vi "SiPM_IV_Tests.vi"(0 "Nb of Pixels":u16, 2 "SiPM Model":string="Hamamatsu_", 3 "SiPM Supplier":string="Hamamatsu_", 4 "Save Reults to file":bool, 5 "Specify folder to save results":path=path "C:/Users/John/Desktop/RESULTS") -> ()   [LabVIEW 2015]
uses:
  <vilib>/Utility/file.llb/Write Delimited Spreadsheet (string).vi
  <vilib>/Utility/file.llb/Write Delimited Spreadsheet (DBL).vi
  <vilib>/Analysis/NI_AALPro.lvlib
panel:
  out "Quenching Resistance":dbl format="%#.3p"
  in  "Process Stop Button":bool
  in  "Read\nTemperature":bool
  in  "Load file":bool
  out "Meassurement \n   In Progress":bool
  out "BIAS Voltage":dbl
  out "Resistance (Overall)":dbl format="%#.3p"
  in  "Start IV":bool
  in  "Current Limit (A)":dbl=0.5
  in  "Enable Time Delay":bool=TRUE
  in  "Time Delay (s)":dbl=1.0
  in  "Nb of Steps":dbl
  in  "Step size (V)":dbl
  in  "Starting Voltage (V)":dbl
  out "I-V graph":cluster{dbl[], "Best Linear Fit":dbl[]}[](graph)
  out "Current Chart":dbl(graph)
  out "Temperature":dbl(slide) scale=0.0..30.0
  in  "Initial Range":dbl=2e-06 min=2e-11 max=0.02 format="%.2e"
  in  "V-Source Range (100:0)":u16(ring)=1 items=["+/- 100 Volts", "+/- 1000 Volts"]
  # "NCSR  DEMOKRITOS\nInstitute of Nuclear and Particle Physics\nDetectors Instrumentation Laboratory"
  # "Si PhotoMultiplier  I-V Measurements"
  # "Device Under Test Type"
  # "Measurement Parameters"
  # "Keithley 6517A"
  # "Additional Parameters"
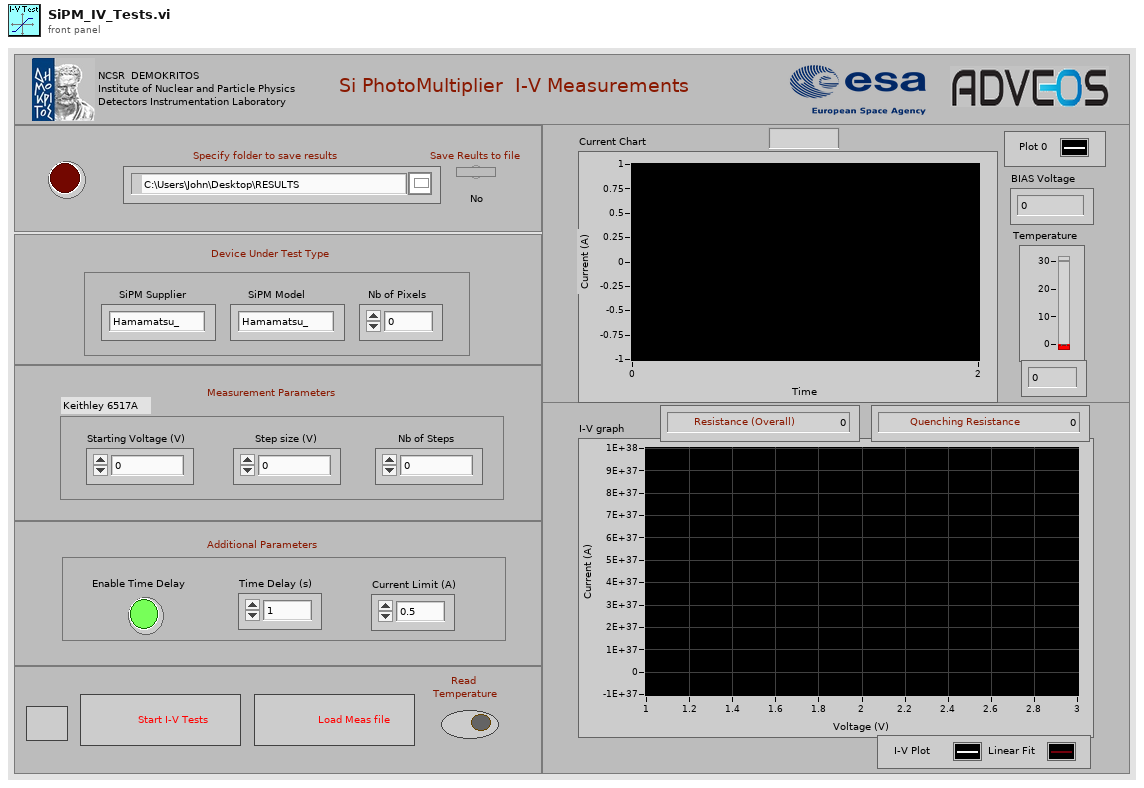
[diagram p1: front panel]
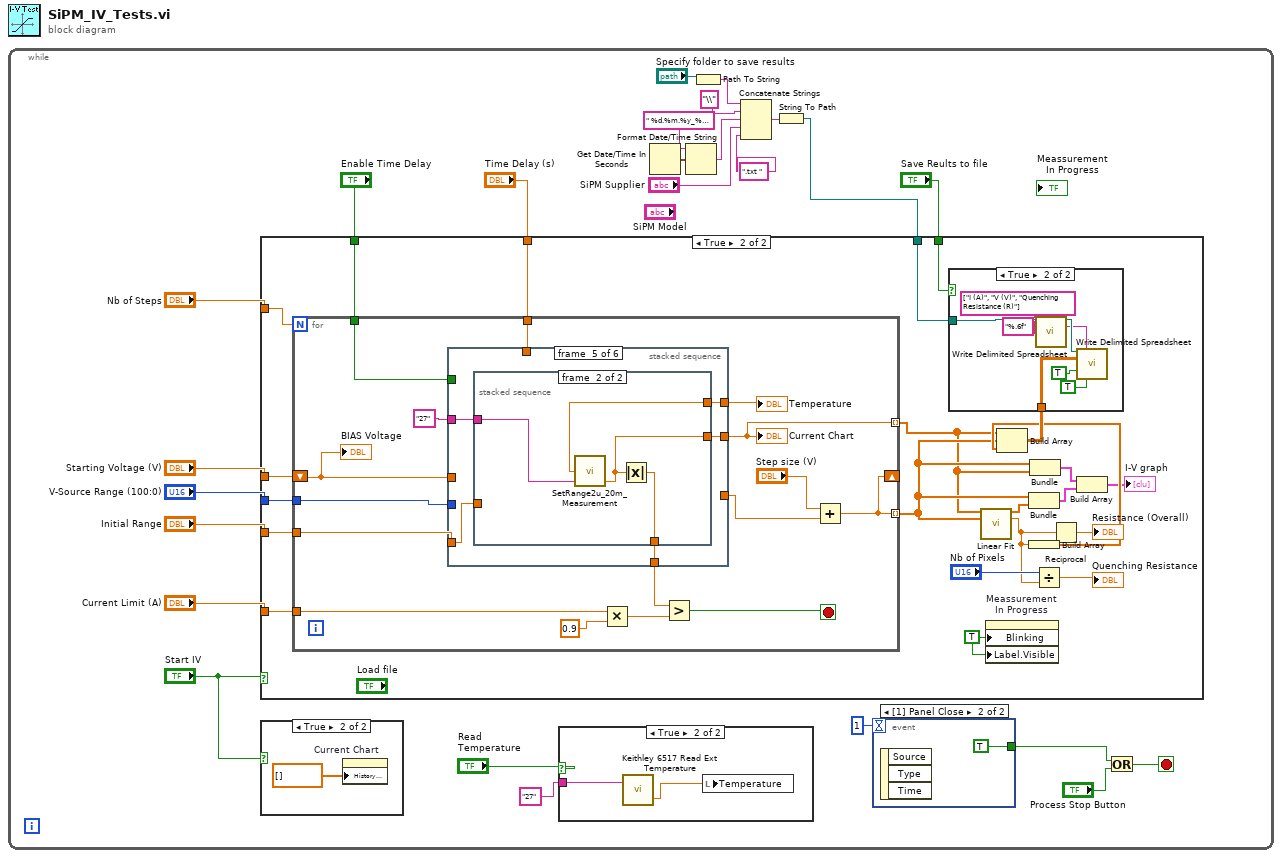
[diagram p0: block diagram]
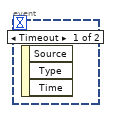
[diagram p2: hidden frame]
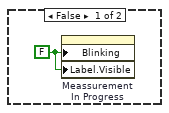
[diagram p3: hidden frame]
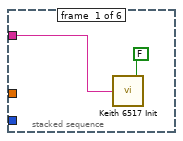
[diagram p5: hidden frame]
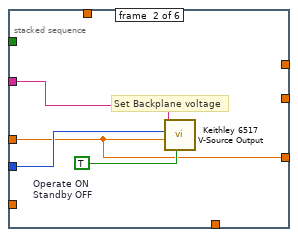
[diagram p6: hidden frame]
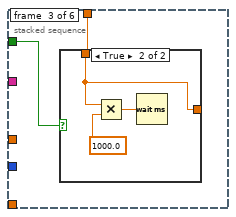
[diagram p7: hidden frame]
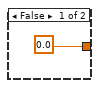
[diagram p8: hidden frame]
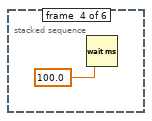
[diagram p9: hidden frame]
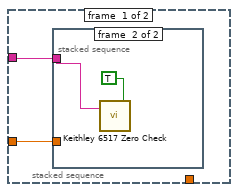
[diagram p10: hidden frame]
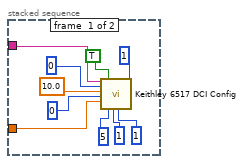
[diagram p11: hidden frame]
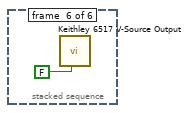
[diagram p12: hidden frame]
diagram:
  n1 = while {
    stop <- w2 stop-if-true
    n2 = case shown="True" "Start IV" {
      frame False {
      }
      frame True {
        n3 = property on="Current Chart" class="WFChart (strict)"("History Data"=dbl[] []) -> ()  [unwired: 2 in, 2 out]
      }
    }
    n4 = case shown="True" "Read\nTemperature" {
      tunnel: "27" ("GPIB address") -> [_ w111]
      frame False {
      }
      frame True {
        n5 = call "Keithley 6517 Read Ext Temperature.vi"("GPIB address"=w111) -> ("External Temperature"=w112:dbl)  [unwired: 1 in, 1 out]
        n6 = local write "Temperature"(w112) -> ()
      }
    }
    n7 = Get Date/Time In Seconds() -> (seconds since 1Jan1904=w14:timestamp)
    n8 = Format Date/Time String(time format string (%c)=" %d.%m.%y_%H.%M_", seconds (now)=w14) -> (date/time string=w9:string)  [unwired: 1 in]
    n9 = Path To String(path="Specify folder to save results") -> (string=w8:string)
    n10 = Concatenate Strings(w8, "\\" ("string"), w9, "SiPM Supplier", ".txt " ("String")) -> (w6:string)
    n11 = String To Path(string=w6) -> (path=w5:path)
    n12 = case shown="True" "Start IV" {
      tunnel: "V-Source Range (100:0)" -> [_ w49]
      tunnel: "Initial Range" -> [_ w48]
      tunnel: "Time Delay (s)" -> [_ w47]
      tunnel: "Enable Time Delay" -> [_ w46]
      tunnel: "Nb of Steps" -> [_ w45]
      tunnel: "Starting Voltage (V)" -> [_ w44]
      tunnel: "Current Limit (A)" -> [_ w43]
      tunnel: "Save Reults to file" -> [_ w39]
      tunnel: w5 -> [_ w38]
      frame False {
        w27 = FALSE ("Blinking")
        n13 = property on="Meassurement \n   In Progress" class="Bool (strict)"("Blinking"=w27, "Label.Visible"=w27) -> ()  [unwired: 2 in, 2 out]
      }
      frame True {
        w33 = TRUE ("Blinking")
        n14 = for {
          N: w45 -> [_]
          tunnel: w49 -> [w71]
          tunnel: w48 -> [w70]
          tunnel: w47 -> [w65]
          tunnel: w46 -> [w64]
          shift-right: [w59] -> _
          shift-left: w44 -> [w57]
          tunnel: w43 -> [w62]
          tunnel: [w59] -> w36 mode=indexing
          tunnel: [w58] -> w29 mode=indexing
          stop <- w63 stop-if-true
          n15 = stacked-sequence {
            tunnel: "27" ("GPIB address\nKeithley 6517") -> [w74 w77 _ _ w90 _]
            tunnel: w71 -> [_ w76 _ _ _ _]
            tunnel: w57 -> [_ w75 _ _ _ _]
            tunnel: w70 -> [_ _ _ _ w89 _]
            tunnel: [_ _ _ _ w88 _] -> w68
            tunnel: [_ _ _ _ w87 _] -> w58
            tunnel: [_ _ _ _ w86 _] -> w66
            tunnel: w64 -> [_ _ w80 _ _ _]
            tunnel: w65 -> [_ _ w79 _ _ _]
            tunnel: [_ w75 _ _ _ _] -> w60
            frame #0 {
              n16 = call "Keith 6517 Init.vi"("Internal Connection"=FALSE, "GPIB address\nKeithley 6517"=w74) -> ()
            }
            frame #1 {
              w78 = TRUE  # Operate ON Standby OFF
              # "Set Backplane voltage"
              n17 = call "Keithley 6517 V-Source Output.vi"("V-Source Operate"=w78, "Output Voltage Value"=w75, "V-Source Range (100:0)"=w76, "GPIB address"=w77) -> ()  [unwired: 6 in, 1 out]
            }
            frame #2 {
              n18 = case shown="True" w80 {
                tunnel: w79 -> [_ w82]
                tunnel: [0.0 w82] -> _
                frame False {
                }
                frame True {
                  n19 = Multiply(x=w82, y=1000.0) -> (x*y=w83:dbl)
                  n20 = Wait (ms)(milliseconds to wait=w83) -> ()  [unwired: 1 out]
                }
              }
            }
            frame #3 {
              n21 = Wait (ms)(milliseconds to wait=100.0) -> ()  [unwired: 1 out]
            }
            frame #4 {
              n22 = stacked-sequence {
                tunnel: w90 -> [w91 w106]
                tunnel: w89 -> [w92 _]
                tunnel: [_ w108] -> w88
                tunnel: [_ w107] -> w87
                tunnel: [_ w105] -> w86
                frame #0 {
                  n23 = stacked-sequence {
                    tunnel: w92 -> [w95 _]
                    tunnel: w91 -> [w94 w103]
                    frame #0 {
                      n24 = call "Keithley 6517 DCI Config.vi"("GPIB address"=w94, "integration time (0:auto)"=0, "NPLC value"=10.0, "range (auto:0)"=0, "range value (amps)"=w95, "damping"=TRUE, "resolution (5.5 digits:4)"=5, "digital filter type (off:0)"=1, "dig. filter count"=1, "filter type control (Moving:0)"=1) -> ()  [unwired: 9 in, 1 out]
                    }
                    frame #1 {
                      n25 = call "Keithley 6517 Zero Check.vi"("Zero Check"=TRUE, "GPIB address"=w103) -> ()  [unwired: 1 in, 1 out]
                    }
                  }
                }
                frame #1 {
                  n26 = call "SetRange2u_20m_Measurement.vi"("GPIB Address"=w106) -> ("Current Measured"=w107:dbl, "External Temperature"=w105:dbl)  [unwired: 1 in, 2 out]
                  n27 = Absolute Value(x=w107) -> (abs(x)=w108:dbl)
                }
              }
            }
            frame #5 {
              n28 = call "Keithley 6517 V-Source Output.vi"("V-Source Operate"=FALSE) -> ()  [unwired: 9 in, 1 out]
            }
          }
          "Current Chart" <- w58
          "Temperature" <- w66
          n29 = Multiply(x=w62, y=0.9) -> (x*y=w67:dbl)
          n30 = Greater?(x=w68, y=w67) -> (0:w63:bool)
          n31 = Add(x="Step size (V)", y=w60) -> (x+y=w59:dbl)
          "BIAS Voltage" <- w57
        }
        n32 = call <vilib>:"Linear Fit.vi"("Y"=w29, "X"=w36) -> ("Best Linear Fit"=w42:dbl[], "slope"=w30:dbl)  [unwired: 9 in, 3 out]
        n33 = property on="Meassurement \n   In Progress" class="Bool (strict)"("Blinking"=w33, "Label.Visible"=w33) -> ()  [unwired: 2 in, 2 out]
        n34 = Bundle(w36, "Best Linear Fit"=w42) -> (w41:cluster{dbl[], "Best Linear Fit":dbl[]})  [unwired: 1 in]
        n35 = Build Array(w30) -> (w37:dbl[])
        n36 = Build Array(w29, w36, w37) -> (w40:dbl[][])
        n37 = case shown="True" w39 {
          tunnel: w40 -> [_ w56]
          tunnel: w38 -> [_ w53]
          frame False {
          }
          frame True {
            n38 = call-poly <vilib>:"Write Delimited Spreadsheet.vi"("file path (dialog if empty)"=w53, "1D data"=string[] ["I (A)", "V (V)", "Quenching Resistance (R)"]) -> ("new file path (Not A Path if cancelled)"=w55:path)  [unwired: 12 in, 1 out]
            n39 = call-poly <vilib>:"Write Delimited Spreadsheet.vi"("file path (dialog if empty)"=w55, "format (%.3f)"="%.6f", "2D data"=w56, "append to file? (F)"=TRUE, "transpose? (F)"=TRUE) -> ()  [unwired: 9 in, 2 out]
          }
        }
        n40 = Bundle(w36, w29) -> (w35:cluster{dbl[], dbl[]})  [unwired: 1 in]
        n41 = Divide(x="Nb of Pixels", y=w30) -> (x/y=→"Quenching Resistance":dbl)
        n42 = Reciprocal(x=w30) -> (1/x=→"Resistance (Overall)":dbl)
        n43 = Build Array(w35, w41) -> (→"I-V graph":cluster{dbl[], "Best Linear Fit":dbl[]}[])
      }
    }
    n44 = event shown="[1] Panel Close" {
      selector: _ -> [_ _]
      dyn-events: _ -> [_ _]
      timeout: 1 -> [_ _]
      tunnel: [_ TRUE ("x")] -> w1
      event Timeout {
        n45 = event-data() -> ()  [unwired: 1 in, 3 out]
      }
      event Panel Close {
        n46 = event-data() -> ()  [unwired: 1 in, 3 out]
      }
    }
    n47 = Or(x=w1, y="Process Stop Button") -> (x .or. y?=w2:bool)
  }
